vi "DFD Probe Check NStage MRate Filter.vi"(1 "multirate filters in":T1[](array[typedef]) {"mMRate_SumWl" min=1 max=32 step=1; "mMRate_InputIwl" min=1 max=32 step=1; "mMRate_GainWl" min=1 max=32 step=1; "mMRate_OutputWl" min=1 max=32 step=1; "mMRate_InputWl" min=1 max=32 step=1; "mMRate_CoefWl" min=1 max=32 step=1; "mMRate_Mode" items=["Default"=-1, "No Rate Change"=0, "Interpolation"=1, "Decimation"=2, "Interpolated"=3, "Rational"=4]}) -> (0 "Boolean":bool)   [LabVIEW 2017, in "NI_DigFilterLicensed.lvlib"]
uses:
  <vilib>/addons/Digital Filter Design/NI_DigFilterLicensed.lvlib
  <vilib>/addons/Digital Filter Design/_Objects.llb/DFD Multirate Filter Obj.ctl
  <vilib>/addons/Digital Filter Design/_Objects.llb/DFD Multirate Mode.ctl
  <vilib>/addons/Digital Filter Design/_Objects.llb/DFD Coef Norm Type.ctl
  <vilib>/addons/Digital Filter Design/_Objects.llb/DFD Round-off Mode.ctl
  <vilib>/addons/Digital Filter Design/_Objects.llb/DFD FXP MRate Multiply Mode.ctl
panel:
  in  "Tab Control":enum32{"Basic Info", "Magnitude Response"}(tab)
  out "quantized?":bool
  in  "Filter gain":dbl format="%#_8g"
  in  "Filter type":i32(ring)=-1 items=["Invalid"=-1, "No Rate Change"=0, "Interpolation"=1, "Decimation"=2]
  in  "Filter factor":i32 min=2
  in  "Number of stages":i32 min=1 max=1 step=1
  in  "Subfactors":i32[](array[numeric]) min=1 step=1
  out "Freq Resp":cluster{"f0":dbl, "df":dbl, "values":dbl[]}[](graph)
  in  "Magnitude in dB":bool=TRUE
  # "Quantized?"
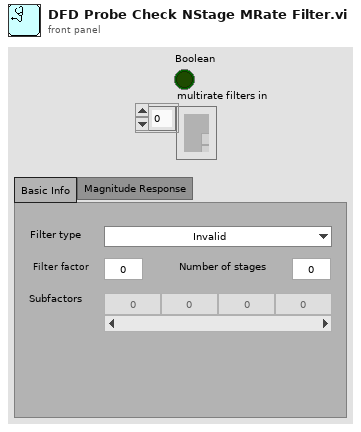
[diagram p1: front panel]
types:
  T1 = typedef "NI_DigFilterLicensed.lvlib/DFD Multirate Filter Obj.ctl" = cluster{"mMRate_Structure":enum16{"CIC", "FIR", "IIR", "Lattice"}, "mMRate_Mode":T2, "mMRate_Factor":i32, "mMRate_FIRParams":cluster{"mMRate_FIR_H":dbl[], "mMRate_FIR_IsNyquist?":bool, "mMRate_FIR_IsSymmetric?":bool}, "mMRate_CICParams":cluster{"mMRate_CIC_#Stage":i32, "mMRate_CIC_Lag":i32, "mMRate_CIC_Type":enum16{"Lowpass", "Highpass"}}, "mMRate_Order":i32, "mMRate_Version":string, "mMRate_Comments":string, "mMRate_RationalFactor":cluster{"mMRate_L":i32, "mMRate_M":i32}, "mMRate_Fs":dbl, "mMRate_Quantized?":bool, "mMRate_QFilterGain":dbl, "mMRate_CoefWl":i16, "mMRate_Scaling":cluster{"mMRate_ScaleByPowerOf2?":bool, "mMRate_ScaleType":T3}, "mMRate_InputWl":i16, "mMRate_OutputWl":i16, "mMRate_OutputMode":T4, "mMRate_MultMode":T5, "mMRate_BitPruning":bool, "mMRate_GainWl":i16, "mMRate_OutputFwl":i16, "mMRate_SumIwl":i16, "mMRate_InputIwl ":i16, "mMRate_SumWl":i16, "mMRate_CoefIwl":i16}
  T2 = typedef "NI_DigFilterLicensed.lvlib/DFD Multirate Mode.ctl" = i16
  T3 = typedef "NI_DigFilterLicensed.lvlib/DFD Coef Norm Type.ctl" = enum16{"No Norm", "Time Domain 1-Norm", "Time Domain 2-Norm", "Time Domain Inf-Norm"}
  T4 = typedef "NI_DigFilterLicensed.lvlib/DFD Round-off Mode.ctl" = enum16{"Nearest", "Truncation"}
  T5 = typedef "NI_DigFilterLicensed.lvlib/DFD FXP MRate Multiply Mode.ctl" = enum16{"Truncated", "Full"}
  T6 = enum8{"Enabled", "Disabled", "Disabled and Grayed Out"}
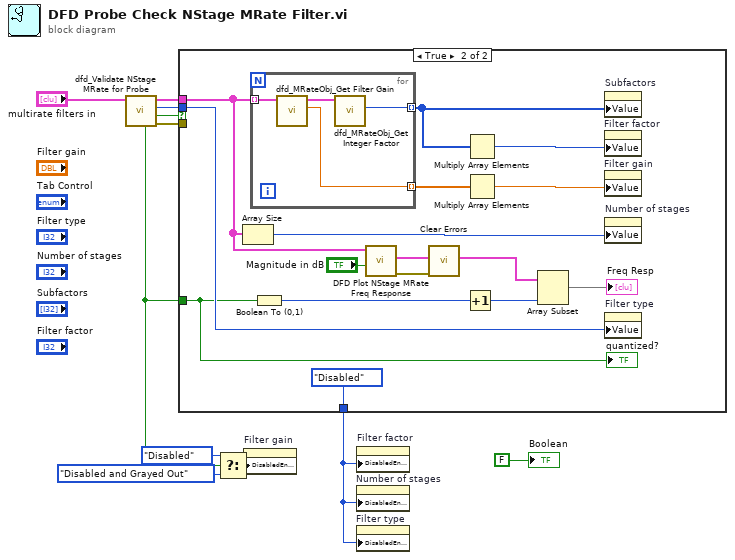
[diagram p0: block diagram]
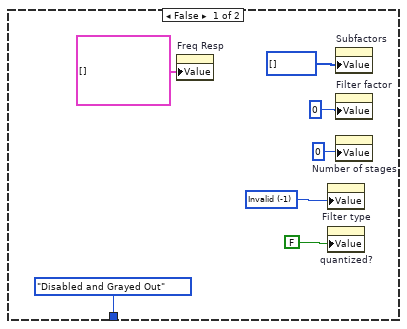
[diagram p2: hidden frame]
diagram:
  n1 = call <vilib>:"dfd_Validate NStage MRate for Probe.vi"("multirate filters in"="multirate filters in") -> ("error out"=w6:errorcluster, "valid?"=w7:bool, "mode"=w9:T2, "multirate filters out"=w10:T1[], "is FXP?"=w5:bool)  [unwired: 6 in]
  n2 = case shown="True" w7 {
    tunnel: w10 -> [_ w24]
    tunnel: w9 -> [_ w33]
    tunnel: w6 -> [_ _]
    tunnel: w5 -> [_ w20]
    tunnel: [T6."Disabled and Grayed Out" ("Disabled") T6."Disabled" ("Disabled")] -> w3
    frame False {
      w16 = -1 items=["Invalid"=-1, "No Rate Change"=0, "Interpolation"=1, "Decimation"=2] ("Filter type")
      n3 = property on="Freq Resp" class="WFGraph (strict)"("Value"=cluster{"f0":dbl, "df":dbl, "values":dbl[]}[] [] ("Freq Resp")) -> ()  [unwired: 2 in, 2 out]
      n4 = property on="Filter type" class="Ring (strict)"("Value"=w16) -> ()  [unwired: 2 in, 2 out]
      n5 = property on="quantized?" class="Bool (strict)"("Value"=FALSE ("quantized?")) -> ()  [unwired: 2 in, 2 out]
      n6 = property on="Subfactors" class="Arr (strict)"("Value"=i32[] [] ("Subfactors")) -> ()  [unwired: 2 in, 2 out]
      n7 = property on="Filter factor" class="DigNum (strict)"("Value"=0 ("Filter factor")) -> ()  [unwired: 2 in, 2 out]
      n8 = property on="Number of stages" class="DigNum (strict)"("Value"=0 ("Number of stages")) -> ()  [unwired: 2 in, 2 out]
    }
    frame True {
      n9 = Array Size(array=w24) -> (size(s)=w21:i32)
      n10 = for {
        tunnel: w24 -> [w34] mode=indexing
        tunnel: [w37] -> w32 mode=indexing
        tunnel: [w35] -> w29 mode=indexing
        n11 = call <vilib>:"dfd_MRateObj_Get Filter Gain.vi"("multirate filter in"=w34) -> ("gain"=w37:dbl, "dup multirate filter"=w36:T1)  [unwired: 9 out]
        n12 = call <vilib>:"dfd_MRateObj_Get Integer Factor.vi"("multirate filter in"=w36) -> ("factor"=w35:i32)  [unwired: 10 out]
      }
      n13 = Boolean To (0,1)(Boolean=w20) -> (0, 1=w27:i16)
      n14 = call <vilib>:"DFD Plot NStage MRate Freq Response.vi"("dB on? (T)"="Magnitude in dB", "multirate filters in"=w24) -> ("error out"=w22:errorcluster, "magnitude responses"=w25:cluster{"f0":dbl, "df":dbl, "values":dbl[]}[])  [unwired: 5 in, 3 out]
      n15 = call <vilib>:"Clear Errors.vi"("error in (no error)"=w22) -> ()  [unwired: 1 in, 6 out]
      n16 = Increment(x=w27) -> (x+1=w26:i16)
      n17 = Multiply Array Elements(1:w29) -> (0:w30:i32)
      n18 = Multiply Array Elements(1:w32) -> (0:w31:dbl)
      n19 = Array Subset(array=w25, length=w26) -> (→"Freq Resp":cluster{"f0":dbl, "df":dbl, "values":dbl[]}[])  [unwired: 1 in]
      n20 = property on="Subfactors" class="Arr (strict)"("Value"=w29) -> ()  [unwired: 2 in, 2 out]
      n21 = property on="Filter factor" class="DigNum (strict)"("Value"=w30) -> ()  [unwired: 2 in, 2 out]
      n22 = property on="Filter gain" class="DigNum (strict)"("Value"=w31) -> ()  [unwired: 2 in, 2 out]
      n23 = property on="Number of stages" class="DigNum (strict)"("Value"=w21) -> ()  [unwired: 2 in, 2 out]
      n24 = property on="Filter type" class="Ring (strict)"("Value"=w33) -> ()  [unwired: 2 in, 2 out]
      "quantized?" <- w20
    }
  }
  n25 = Select(t=T6."Disabled" ("Disabled"), s=w5, f=T6."Disabled and Grayed Out" ("Disabled")) -> (s? t:f=w4:T6)
  n26 = property on="Filter gain" class="DigNum (strict)"("DisabledEnum"=w4) -> ()  [unwired: 2 in, 2 out]
  n27 = property on="Filter factor" class="DigNum (strict)"("DisabledEnum"=w3) -> ()  [unwired: 2 in, 2 out]
  n28 = property on="Number of stages" class="DigNum (strict)"("DisabledEnum"=w3) -> ()  [unwired: 2 in, 2 out]
  n29 = property on="Filter type" class="Ring (strict)"("DisabledEnum"=w3) -> ()  [unwired: 2 in, 2 out]
  "Boolean" <- FALSE ("Boolean")
